vi "题目二的子vi.vi"() -> ()   [LabVIEW 2017]
panel:
  out "数值":i32
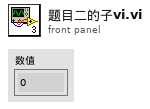
[diagram p1: front panel]
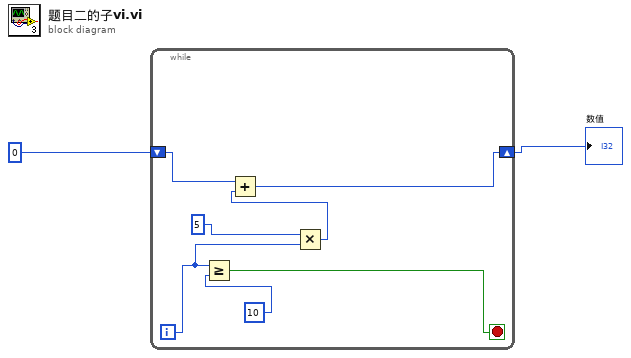
[diagram p0: block diagram]
diagram:
  n1 = while {
    shift-right: [w7] -> w1
    shift-left: 0 -> [w9]
    i -> [w5]
    stop <- w6 stop-if-true
    n2 = Greater Or Equal?(x=w5, y=10) -> (x >= y?=w6:bool)
    n3 = Multiply(x=5, y=w5) -> (x*y=w3:i32)
    n4 = Add(x=w9, y=w3) -> (x+y=w7:i32)
  }
  "数值" <- w1
